vi "CoordAxis_New.vi"(9 "Z":dbl, 10 "Y":dbl, 11 "X":dbl) -> (3 "out Coordinate Axis":T1)   [LabVIEW 2019, in "Trajectory_Library.lvlib"]
doc: "Convenience constructors that takes in x and y values directly instead of having to construct a Translation2d.\n\nParameters:\n - X- The x component of the translational component of the pose.\n - Y - The y component of the translational component of the pose.\n - Rotation (Heading) - The rotational component of the pose.\n\nReturns:\n - OUT POSE - Output POSE"
uses:
  Trajectory_Library.lvlib
  COORDINATE_AXIS.ctl
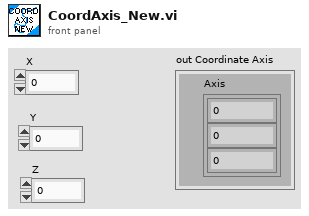
[diagram p1: front panel]
types:
  T1 = typedef "Trajectory_Library.lvlib/COORDINATE_AXIS.ctl" = cluster{"Axis":dbl[]}
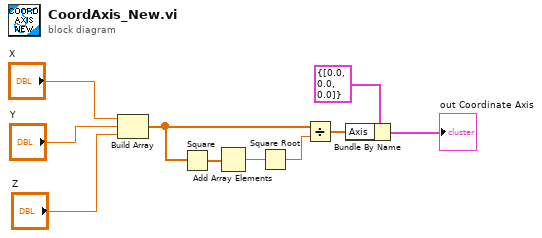
[diagram p0: block diagram]
diagram:
  n1 = Build Array("X", "Y", "Z") -> (w4:dbl[])
  n2 = Square(x=w4) -> (x^2=w3:dbl[])
  n3 = Add Array Elements(numeric array=w3) -> (sum=w2:dbl)
  n4 = Square Root(x=w2) -> (sqrt(x)=w1:dbl)
  n5 = Divide(x=w4, y=w1) -> (x/y=w6:dbl[])
  n6 = Bundle By Name(cluster=T1 {"Axis"=[0.0, 0.0, 0.0]} ("sumPOSE"), "Axis"=w6) -> (→"out Coordinate Axis":T1)
